vi "Device Control Panel.vi"(8 "error in (no error)":errorcluster, 11 "Class":refnum<class "Device.lvclass">) -> (0 "error out":errorcluster, 3 "Class out":refnum<class "Device.lvclass">)   [LabVIEW 2015, in "Device.lvclass"]
uses:
  Device.lvclass
  Device.lvclass/Device.ctl
panel:
  in  "Data":cluster{"Nothing to configure":string}
  out "Device Name":string
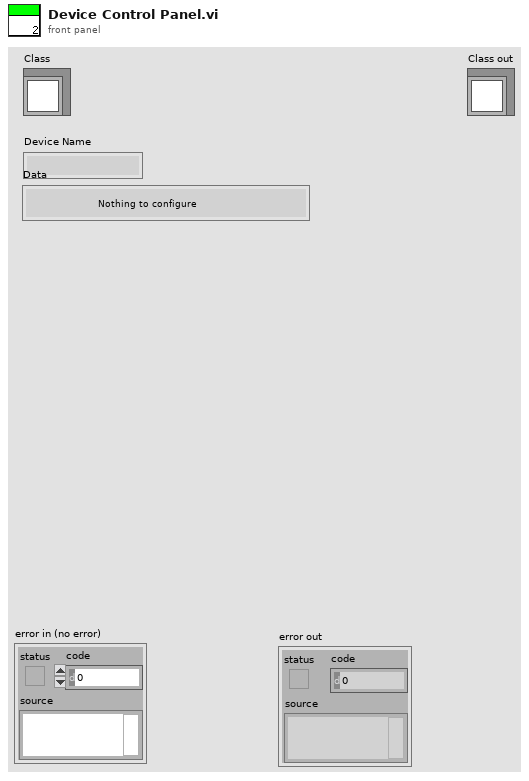
[diagram p1: front panel]
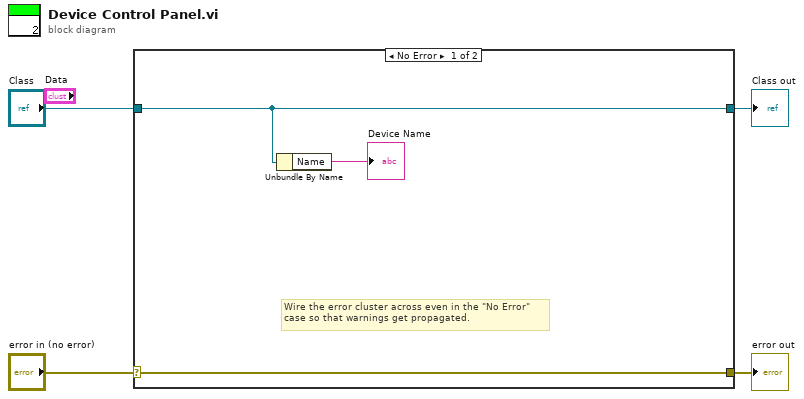
[diagram p0: block diagram]
diagram:
  n1 = case shown="No Error" "error in (no error)" {
    selector: "error in (no error)" -> [w7 w9]
    tunnel: [w7 w9] -> w3
    tunnel: [w6 w8] -> w1
    tunnel: "Class" -> [w6 w8]
    frame No Error {
      # "Wire the error cluster across even in the \"No Error\"\ncase so that warnings get propagated."
      n2 = Unbundle By Name(w6) -> ("Name"=→"Device Name":string)
    }
    frame Error {
    }
  }
  "error out" <- w3
  "Class out" <- w1
